vi "Client Connection Loop.vi"(8 "error in (no error)":errorcluster, 11 "TCPMessaging in":refnum<class "TCPMessaging.lvclass">) -> (0 "error out":errorcluster)   [LabVIEW 2020, in "Vecto.lvlib" / "TCPMessaging.lvclass"]
uses:
  TCPMessaging.lvclass
  TCPMessaging.lvclass/TCPMessaging.ctl
  proto/TcpClientHello/TcpClientHello.lvlib
  Connection State.ctl
  Vecto.lvlib
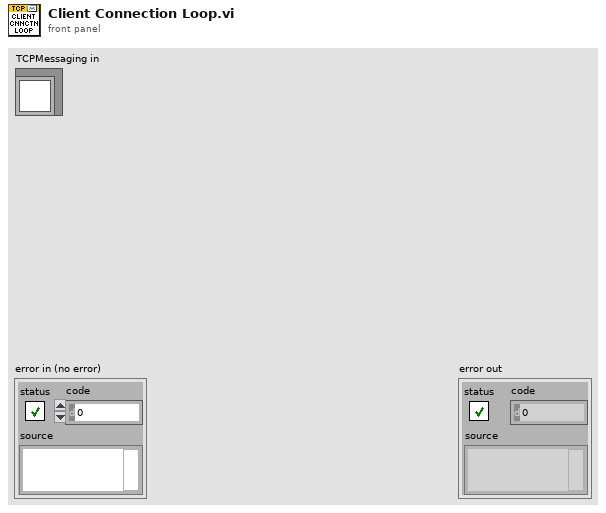
[diagram p1: front panel]
types:
  T1 = typedef "Vecto.lvlib/Connection State.ctl" = enum16{"Connected", "Disconnected"}
  T2 = typedef "TcpClientHello.lvlib/Data.ctl" = cluster{"node_id":u32, "system":string, "cluster":string, "node_name":string, "app_version":string, "config_version":string}
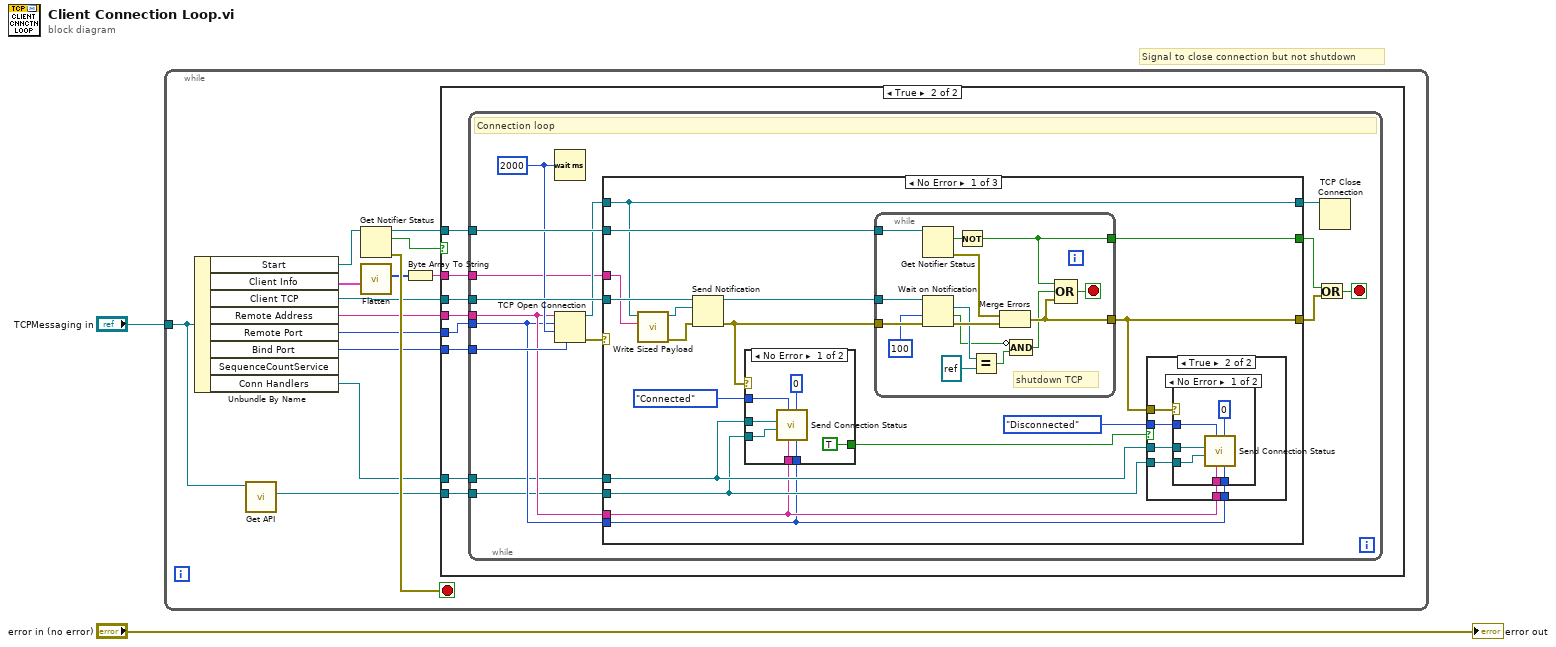
[diagram p0: block diagram]
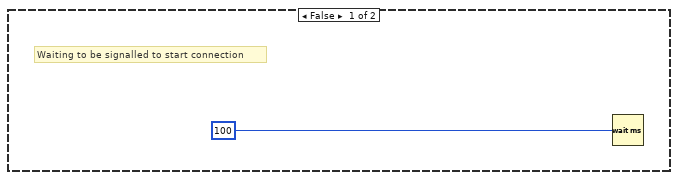
[diagram p2: hidden frame]
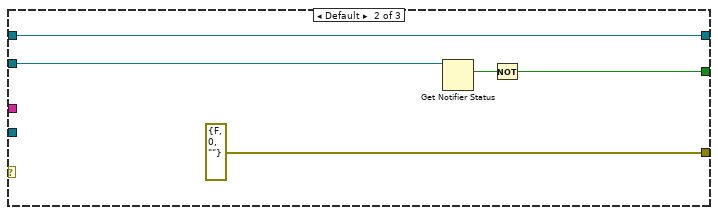
[diagram p6: hidden frame]
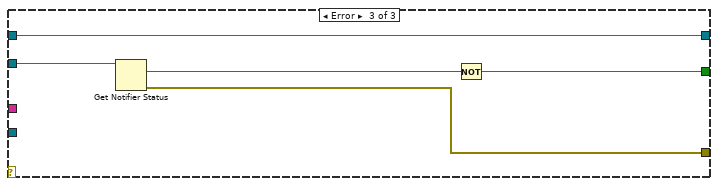
[diagram p7: hidden frame]
diagram:
  # "Signal to close connection but not shutdown"
  n1 = while {
    tunnel: "TCPMessaging in" -> [w4]
    stop <- w16 stop-if-true
    n2 = Unbundle By Name(w4) -> ("Start"=w10:refnum<notifier>, "Client Info"=w8:T2, "Client TCP"=w9:refnum<notifier>, "Remote Address"=w15:string, "Remote Port"=w14:u16, "Bind Port"=w11:u16, "Conn Handlers"=w5:refnum<queue>)  [unwired: 1 out]
    n3 = call "Get API.vi"("TCPMessaging in"=w4) -> ("TCP Messaging API"=w3:refnum<class "TCPMessageAPI.lvclass">)  [unwired: 8 in, 2 out]
    n4 = Get Notifier Status(notifier=w10) -> (notifier out=w13:refnum<notifier>, current notification=w12:bool, error out=w16:errorcluster)  [unwired: 1 in, 2 out]
    n5 = call "Flatten.vi"("Data"=w8) -> ("Buffer"=w7:u8[])  [unwired: 9 in, 1 out]
    n6 = Byte Array To String(unsigned byte array=w7) -> (string=w6:string)
    n7 = case shown="True" w12 {
      tunnel: w15 -> [_ w22]
      tunnel: w14 -> [_ w23]
      tunnel: w13 -> [_ w25]
      tunnel: w11 -> [_ w24]
      tunnel: w9 -> [_ w21]
      tunnel: w6 -> [_ w20]
      tunnel: w5 -> [_ w19]
      tunnel: w3 -> [_ w18]
      frame False {
        # "Waiting to be signalled to start connection"
        n8 = Wait (ms)(milliseconds to wait=u32 100) -> ()  [unwired: 1 out]
      }
      frame True {
        n9 = while {
          tunnel: w25 -> [w36]
          tunnel: w24 -> [w39]
          tunnel: w23 -> [w28]
          tunnel: w22 -> [w29]
          tunnel: w21 -> [w37]
          tunnel: w20 -> [w30]
          tunnel: w19 -> [w27]
          tunnel: w18 -> [w26]
          stop <- w40 stop-if-true
          w31 = 2000 ("timeout ms (60000)")
          # "Connection loop"
          n10 = Wait (ms)(milliseconds to wait=w31) -> ()  [unwired: 1 out]
          n11 = TCP Open Connection(address=w29, remote port or service name=w28, timeout ms (60000)=w31, local port=w39) -> (connection ID=w33:refnum<k5>, error out=w38:errorcluster)  [unwired: 1 in]
          n12 = case shown="No Error" w38 {
            tunnel: w33 -> [w52 w95 w98]
            tunnel: w37 -> [w56 _ _]
            tunnel: w36 -> [w57 w94 w101]
            tunnel: [w42 errorcluster {"status"=FALSE, "code"=0, "source"=""} ("error IO") w97] -> w35
            tunnel: [w54 w92 w99] -> w34
            tunnel: [w52 w95 w98] -> w32
            tunnel: w30 -> [w53 _ _]
            tunnel: w29 -> [w44 _ _]
            tunnel: w28 -> [w43 _ _]
            tunnel: w27 -> [w46 _ _]
            tunnel: w26 -> [w45 _ _]
            frame No Error {
              n13 = call "Write Sized Payload.vi"("Payload"=w53, "TCP in"=w52) -> ("error out"=w50:errorcluster, "TCP"=w51:refnum<k5>)  [unwired: 8 in]
              n14 = Send Notification(notification=w51, notifier=w56, error in (no error)=w50) -> (notifier out=w55:refnum<notifier>, error out=w49:errorcluster)
              n15 = case shown="No Error" w49 {
                tunnel: w46 -> [w64 _]
                tunnel: w45 -> [w63 _]
                tunnel: w44 -> [w62 _]
                tunnel: w43 -> [w61 _]
                tunnel: Connection_State."Connected" ("State") -> [w60 _]
                tunnel: [TRUE _] -> w41
                frame No Error {
                  n16 = call "Send Connection Status.vi"("Port"=w61, "Node ID"=u32 0, "Address"=w62, "State"=w60, "TCPMessageAPI"=w63, "Conn Handlers"=w64) -> ()  [unwired: 6 in]
                }
                frame Error {
                }
              }
              n17 = while {
                tunnel: w57 -> [w75]
                tunnel: w55 -> [w74]
                tunnel: [w68] -> w54
                tunnel: [w78] -> w42
                tunnel: w49 -> [w79]
                stop <- w67 stop-if-true
                # "shutdown TCP"
                n18 = Get Notifier Status(notifier=w75) -> (current notification=w76:bool, error out=w70:errorcluster)  [unwired: 1 in, 3 out]
                n19 = Wait on Notification(notifier=w74, timeout in ms (-1)=100, error in (no error)=w79) -> (notification=w72:refnum<k5>, timed out?=w65:bool, error out=w77:errorcluster)  [unwired: 1 in, 1 out]
                n20 = Not(x=w76) -> (.not. x?=w68:bool)
                n21 = Equal?(x=w72, y=refnum<k5> refnum) -> (x = y?=w69:bool)
                n22 = Merge Errors(w70, w77) -> (w78:errorcluster)
                n23 = Compound Arithmetic op=AND(invert w65, w69) -> (w66:bool)
                n24 = Compound Arithmetic op=OR(w68, w66, w78) -> (w67:bool)
              }
              n25 = case shown="True" w41 {
                tunnel: Connection_State."Disconnected" ("State") -> [_ w85]
                tunnel: w46 -> [_ w84]
                tunnel: w45 -> [_ w83]
                tunnel: w44 -> [_ w82]
                tunnel: w43 -> [_ w81]
                tunnel: w42 -> [_ w80]
                frame False {
                }
                frame True {
                  n26 = case shown="No Error" w80 {
                    tunnel: w84 -> [w91 _]
                    tunnel: w83 -> [w90 _]
                    tunnel: w82 -> [w89 _]
                    tunnel: w81 -> [w88 _]
                    tunnel: w85 -> [w87 _]
                    frame No Error {
                      n27 = call "Send Connection Status.vi"("Port"=w88, "Node ID"=u32 0, "Address"=w89, "State"=w87, "TCPMessageAPI"=w90, "Conn Handlers"=w91) -> ()  [unwired: 6 in]
                    }
                    frame Error {
                    }
                  }
                }
              }
            }
            frame Default {
              n28 = Get Notifier Status(notifier=w94) -> (current notification=w93:bool)  [unwired: 1 in, 4 out]
              n29 = Not(x=w93) -> (.not. x?=w92:bool)
            }
            frame Error {
              n30 = Get Notifier Status(notifier=w101) -> (current notification=w100:bool, error out=w97:errorcluster)  [unwired: 1 in, 3 out]
              n31 = Not(x=w100) -> (.not. x?=w99:bool)
            }
          }
          n32 = Or(x=w34, y=w35) -> (x .or. y?=w40:bool)
          n33 = TCP Close Connection(connection ID=w32) -> ()  [unwired: 2 in, 2 out]
        }
      }
    }
  }
  "error out" <- "error in (no error)"
